vi "Message type.vi"(11 "IAbortHandler in":refnum<class "IAbortHandler.lvclass">) -> (2 "Internal message type":T1, 3 "IAbortHandler out":refnum<class "IAbortHandler.lvclass">)   [LabVIEW 2020, in "wamplv.lvlib" / "IAbortHandler.lvclass"]
uses:
  IAbortHandler.lvclass
  TypeDefs/Internal message type.ctl
  wamplv.lvlib
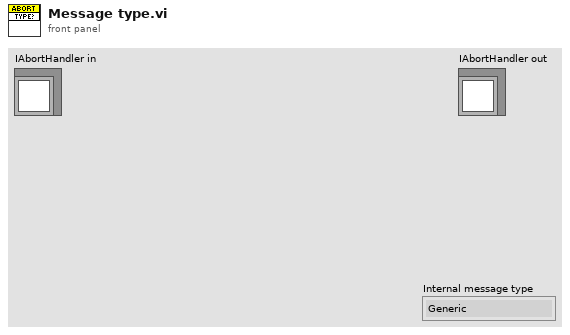
[diagram p1: front panel]
types:
  T1 = typedef "wamplv.lvlib/Internal message type.ctl" = enum16{"Generic", "Generic with write output", "Handle Result", "Handle Error", "Handle Abort"}
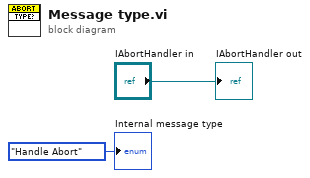
[diagram p0: block diagram]
diagram:
  "IAbortHandler out" <- "IAbortHandler in"
  "Internal message type" <- Internal_message_type."Handle Abort" ("Internal message type")
